vi "MergeOverlay.vi"(7 "Groups":string[](array[string]), 8 "error in":errorcluster, 9 "Color Palette":T1[](array[typedef]), 10 "Dst Reference In":T2, 11 "Src Reference In":T2) -> (0 "error out":errorcluster, 3 "Dst Reference Out":T2)   [LabVIEW 2024, in "OpenLvVision_Overlays.lvlib"]
doc: "This VI embeds a nondestructive overlay directly into the image content, effectively converting it into a destructive (permanent) overlay. Subsequently, the original separate nondestructive overlay is removed. The resulting image is provided in RGB format"
uses:
  OpenLvVision_Overlays.lvlib
  <vilib>/OpenLvVision/OpenLvVision_Image/Management/TypeDef/OLV Image.ctl
  <vilib>/OpenLvVision/OpenLvVision_Image/File/TypeDef/OLV ColorPaletteValue.ctl
  <vilib>/OpenLvVision/OpenLvVision_Image/Management/OLV Management.lvlib
  <vilib>/OpenLvVision/OpenLvVision_Image/File/OLV File.lvlib
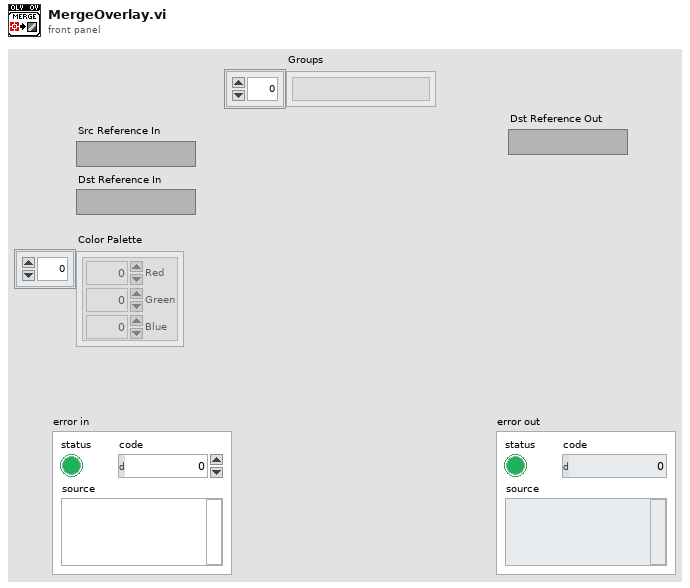
[diagram p1: front panel]
types:
  T1 = typedef "OLV OpenLvVision_Image.lvlib/OLV File.lvlib/OLV ColorPaletteValue.ctl" = cluster{"Red":u8, "Green":u8, "Blue":u8}
  T2 = typedef "OLV OpenLvVision_Image.lvlib/OLV Management.lvlib/OLV Image.ctl" = refnum<image>
  T3 = typedef "IMAQ Image.ctl" = refnum<image>
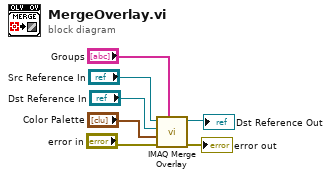
[diagram p0: block diagram]
diagram:
  n1 = call "IMAQ Merge Overlay"("Groups"="Groups", "error in (no error)"="error in", "Color Palette"="Color Palette", "Image Dst"="Dst Reference In", "Image Src"="Src Reference In") -> ("error out"=→"error out":errorcluster, "Image Dst Out"=→"Dst Reference Out":T3)  [unwired: 5 in]
